vi "Search and Replace Inverter Data.vi"(10 "Signal Value in":string[](array[string]), 11 "Signal Name":string[](array[string])) -> (3 "Signal Value out":string[](array[string]))   [LabVIEW 2023, in "HardwareAbstractionLayer_LVOOP.lvlib" / "Report.lvclass"]
uses:
  Report.lvclass
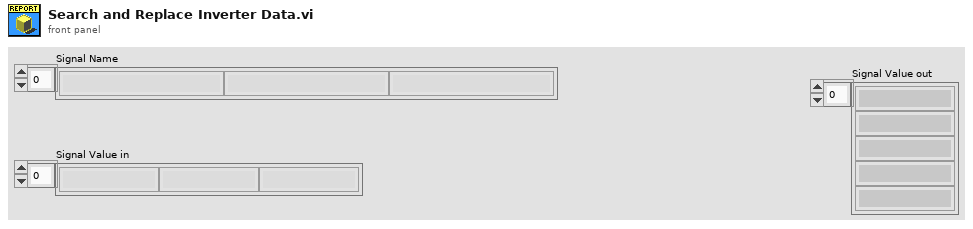
[diagram p1: front panel]
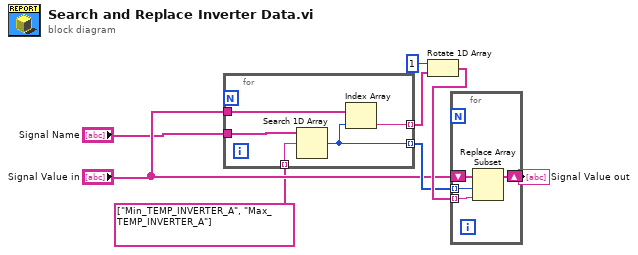
[diagram p0: block diagram]
diagram:
  n1 = for {
    tunnel: "Signal Name" -> [w13]
    tunnel: string[] ["Min_TEMP_INVERTER_A", "Max_TEMP_INVERTER_A"] -> [w12] mode=indexing
    tunnel: "Signal Value in" -> [w11]
    tunnel: [w10] -> w6 mode=indexing
    tunnel: [w9] -> w5 mode=indexing
    n2 = Search 1D Array(1D array=w13, element=w12) -> (index of element=w9:i32)  [unwired: 1 in]
    n3 = Index Array(array=w11, index=w9) -> (element=w10:string)
  }
  n4 = Rotate 1D Array(1:w6, 2:1 ("n")) -> (0:w7:string[])
  n5 = for {
    shift-right: [w16] -> w4
    shift-left: "Signal Value in" -> [w17]
    tunnel: w5 -> [w15] mode=indexing
    tunnel: w7 -> [w14] mode=indexing
    n6 = Replace Array Subset(array=w17, new element=w14, index=w15) -> (w16:string[])
  }
  "Signal Value out" <- w4
